vi "S2C_M2p5942_Proc_MultiPurposeIO.vi"(7 "Local?":bool, 8 "Error In":errorcluster, 10 "Command":string, 11 "JSON String":string) -> (0 "Error Out":errorcluster, 3 "Response":variant)   [LabVIEW 2024]
uses:
  S2C_M2p5942_Proc_Globals.vi
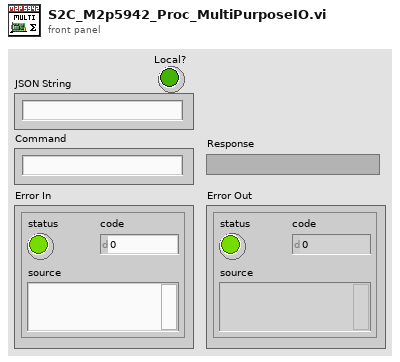
[diagram p1: front panel]
types:
  T1 = cluster{"X0 Mode":u16, "X1 Mode":u16, "X2 Mode":u16, "X3 Mode":u16, "X0 Send":bool, "X1 Send":bool, "X2 Send":bool, "X3 Send":bool, "X1 Trigger Mode":u16, "X2 Trigger Mode":u16, "X3 Trigger Mode":u16, "X1 Pulsewidth":u32, "X2 Pulsewidth":u32, "X3 Pulsewidth":u32, "ASync Read":bool, "ASync Data":i32}
  T2 = cluster{"X0 Mode":u16, "X1 Mode":u16, "X2 Mode":u16, "X3 Mode":u16, "X0 Send":bool, "X1 Send":bool, "X2 Send":bool, "X3 Send":bool, "X1 Trigger Mode":u16, "X2 Trigger Mode":u16, "X3 Trigger Mode":u16, "X1 Pulsewidth":u32, "X2 Pulsewidth":u32, "X3 Pulsewidth":u32, "ASync Read":bool, "ASync":i32, "AI":bool}
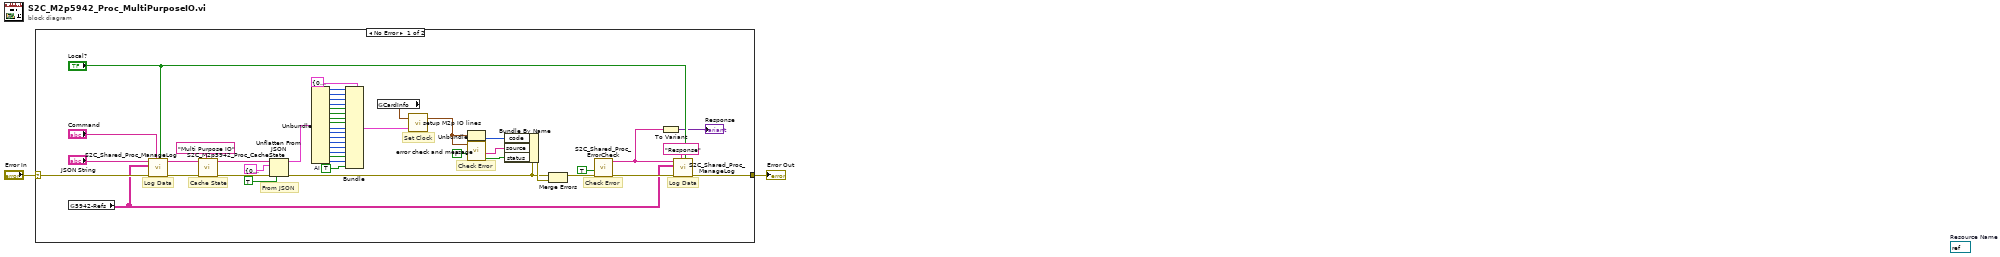
[diagram p0: block diagram]
diagram:
  (unwired) refnum<visa-resource-name> refnum  # Resource Name
  n1 = case shown="No Error" "Error In" {
    selector: "Error In" -> [w48 w50]
    tunnel: [w46 w50] -> w1
    frame No Error {
      w13 = TRUE  # AI
      # "Check Error"
      # "Set Clock"
      # "Check Error"
      # "Cache State"
      # "Log Data"
      # "Log Data"
      # "From JSON"
      n2 = global read "S2C_M2p5942_Proc_Globals.vi" "5942-Refs"() -> (w36:string[][])
      n3 = call "S2C_Shared_Proc_ManageLog.vi"("Local?"="Local?", "Command"="Command", "Error In"=w48, "Refs"=w36, "Data In"="JSON String") -> ("Error Out"=w44:errorcluster, "Data Out"=w43:string)  [unwired: 5 in]
      n4 = call "S2C_M2p5942_Proc_CacheState.vi"("Label"="Multi Purpose IO", "Error In"=w44, "Data In"=w43) -> ("Error Out"=w41:errorcluster, "Data Out"=w42:string)  [unwired: 7 in]
      n5 = Unflatten From JSON(JSON string=w42, type and defaults=T1 {"X0 Mode"=0, "X1 Mode"=0, "X2 Mode"=0, "X3 Mode"=0, "X0 Send"=FALSE, "X1 Send"=FALSE, "X2 Send"=FALSE, "X3 Send"=FALSE, "X1 Trigger Mode"=0, "X2 Trigger Mode"=0, "X3 Trigger Mode"=0, "X1 Pulsewidth"=0, "X2 Pulsewidth"=0, "X3 Pulsewidth"=0, "ASync Read"=FALSE, "ASync Data"=0} ("Mulit-PurpIO"), default null elements? (F)=TRUE, error in (no error)=w41) -> (value=w31:T1, error out=w5:errorcluster)  [unwired: 3 in]
      n6 = Unbundle(w31) -> ("X0 Mode"=w30:u16, "X1 Mode"=w28:u16, "X2 Mode"=w27:u16, "X3 Mode"=w26:u16, "X0 Send"=w25:bool, "X1 Send"=w24:bool, "X2 Send"=w23:bool, "X3 Send"=w22:bool, "X1 Trigger Mode"=w21:u16, "X2 Trigger Mode"=w20:u16, "X3 Trigger Mode"=w19:u16, "X1 Pulsewidth"=w18:u32, "X2 Pulsewidth"=w17:u32, "X3 Pulsewidth"=w16:u32, "ASync Read"=w15:bool, "ASync Data"=w14:i32)
      n7 = Bundle(cluster=T2 {"X0 Mode"=0, "X1 Mode"=0, "X2 Mode"=0, "X3 Mode"=0, "X0 Send"=FALSE, "X1 Send"=FALSE, "X2 Send"=FALSE, "X3 Send"=FALSE, "X1 Trigger Mode"=0, "X2 Trigger Mode"=0, "X3 Trigger Mode"=0, "X1 Pulsewidth"=0, "X2 Pulsewidth"=0, "X3 Pulsewidth"=0, "ASync Read"=FALSE, "ASync"=0, "AI"=FALSE} ("Mulit-PurpIO"), "X0 Mode"=w30, "X1 Mode"=w28, "X2 Mode"=w27, "X3 Mode"=w26, "X0 Send"=w25, "X1 Send"=w24, "X2 Send"=w23, "X3 Send"=w22, "X1 Trigger Mode"=w21, "X2 Trigger Mode"=w20, "X3 Trigger Mode"=w19, "X1 Pulsewidth"=w18, "X2 Pulsewidth"=w17, "X3 Pulsewidth"=w16, "ASync Read"=w15, "ASync"=w14, "AI"=w13) -> (w12:T2)
      n8 = global read "S2C_M2p5942_Proc_Globals.vi" "CardInfo"() -> (w32:cluster{"Card Handle":u64, "Error Code":u32})
      n9 = call "setup M2p IO lines.vi"("Multi Purpose IO Lines"=w12, "Card Info In"=w32) -> ("Card Info Out"=w4:cluster{"Card Handle":u64, "Error Code":u32})  [unwired: 1 in]
      n10 = Unbundle(w4) -> ("Error Code"=w8:u32)  [unwired: 1 out]
      n11 = call "error check and message.vi"("Display Message (true)"=FALSE, "Card Info In"=w4) -> ("Error occurred"=w6:bool, "Error Message"=w7:string)  [unwired: 3 in, 1 out]
      n12 = Bundle By Name(cluster=w5, "code"=w8, "source"=w7, "status"=w6) -> (w10:errorcluster)
      n13 = Merge Errors(w5, w10) -> (w3:errorcluster)
      n14 = call "S2C_Shared_Proc_ErrorCheck.vi"("Error In"=w3, "ExpReply?"=TRUE) -> ("Error Out"=w38:errorcluster, "Status"=w34:string)  [unwired: 8 in]
      n15 = To Variant(anything=w34) -> (Variant=→"Response":variant)
      n16 = call "S2C_Shared_Proc_ManageLog.vi"("Local?"="Local?", "Command"="Response", "Error In"=w38, "Refs"=w36, "Data In"=w34) -> ("Error Out"=w46:errorcluster)  [unwired: 5 in, 1 out]
    }
    frame Error {
    }
  }
  "Error Out" <- w1
